vi "FFT Symbolic.vi"() -> ()   [LabVIEW 2020]
doc: "Calculates the Fourier transform for a symbolic equation that is entered on the front panel."
uses:
  <vilib>/Analysis/2dsp.llb/Real FFT.vi
  <vilib>/gmath/NI_Gmath.lvlib
  <vilib>/Analysis/NI_AALPro.lvlib
panel:
  in  "Tab Control":enum32{"Background", "Example"}(tab)
  out "OK":bool
  in  "Signal Type":u16(ring) items=["Square", "Sine", "Complex", "Arbitrary"]
  out "Response":cluster{"X Values":dbl[], "Y Values":dbl[]}[](graph)
  in  "function":string="square(x)-0.5"
  in  "order":i32(slide)=25 scale=0.0..100.0
  in  "Stop":bool
  # "Overview: Calculates the Fourier transform for a symbolic equation.\nRequirements: LabVIEW Full Development System\nInstructions:\n1. Run the VI and select the Example tab.\n2. Change the Signal Type and verify how this affects the response of the signal.\n3. Increase the order to see how the Gibbs Phenomena influences the signal.\n4. Click Stop to stop the VI."
  # "Gibbs Phenomenon"
  # "Fourier series 5th order"
  # "Fourier series 25th order"
  # "Fourier series can approximate any periodic function.\nThe more elements the better the approximation. The example depicts the approximation of a step function. Certain overshoot values are not avoidable in the case of discontinuous functions."
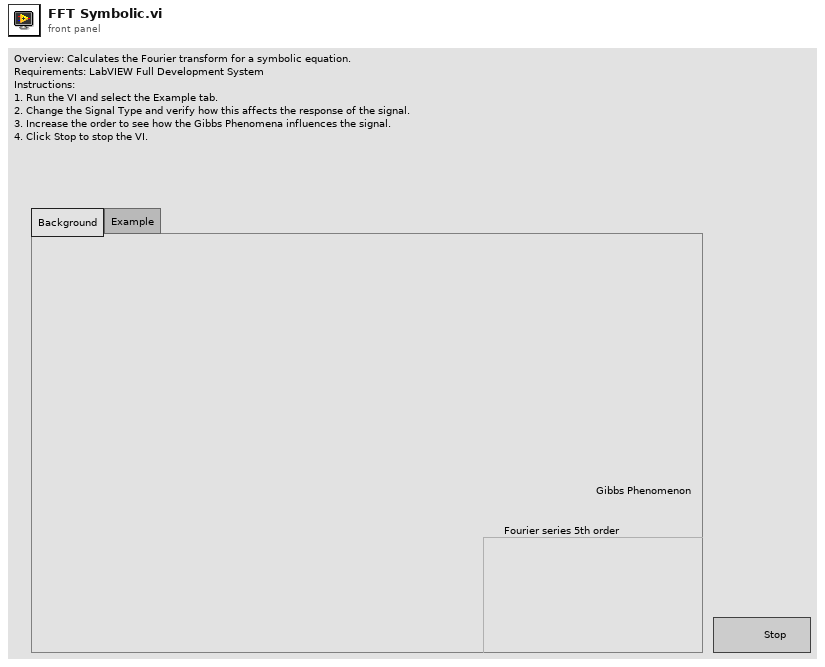
[diagram p1: front panel]
types:
  T1 = enum8{"Enabled", "Disabled", "Disabled and Grayed Out"}
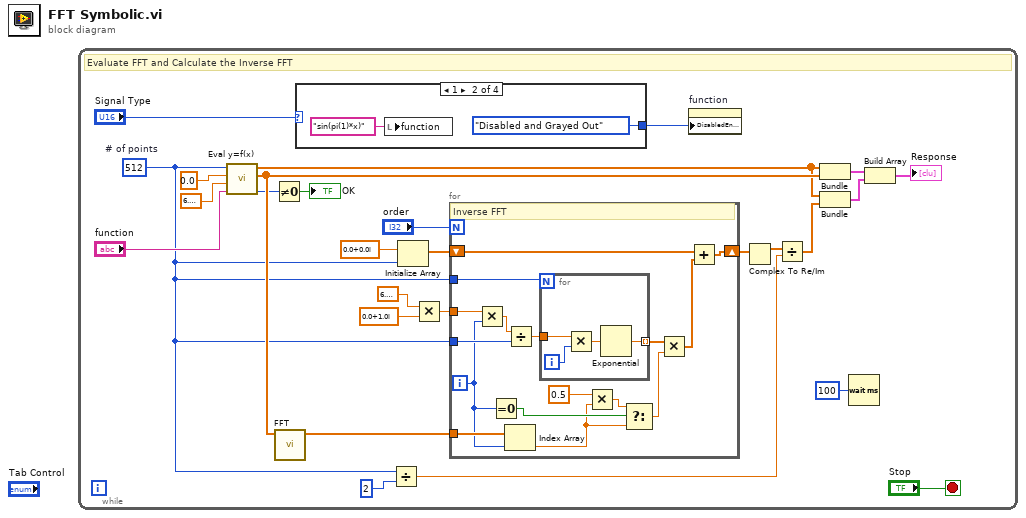
[diagram p0: block diagram]
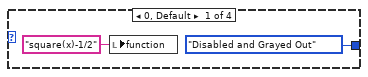
[diagram p2: hidden frame]
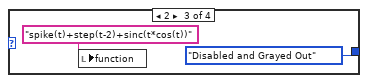
[diagram p3: hidden frame]
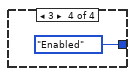
[diagram p4: hidden frame]
diagram:
  n1 = while {
    stop <- "Stop" stop-if-true
    w11 = 512  # # of points
    # "Evaluate FFT and Calculate the Inverse FFT"
    n2 = call <vilib>:"Eval y=f(x).vi"("formula"="function", "end"=6.283185307179586, "start"=0.0, "number of points"=w11) -> ("error"=w7:i32, "Y Values"=w26:dbl[], "X Values"=w19:dbl[])  [unwired: 1 out]
    n3 = Not Equal To 0?(x=w7) -> (x != 0?=→"OK":bool)
    n4 = call-poly <vilib>:"FFT.vi"("X"=w26) -> ("FFT {X}"=w20:cdb[])  [unwired: 2 in, 8 out]
    n5 = case shown="1" "Signal Type" {
      tunnel: [T1."Disabled and Grayed Out" ("Disabled") T1."Disabled and Grayed Out" ("Disabled") T1."Disabled and Grayed Out" ("Disabled") T1."Enabled" ("Disabled")] -> w5
      frame 0, Default {
        n6 = local write "function"("square(x)-1/2" ("function")) -> ()
      }
      frame 1 {
        n7 = local write "function"("sin(pi(1)*x)" ("function")) -> ()
      }
      frame 2 {
        n8 = local write "function"("spike(t)+step(t-2)+sinc(t*cos(t))" ("function")) -> ()
      }
      frame 3 {
      }
    }
    n9 = Divide(x=w11, y=2) -> (x/y=w15:dbl)
    n10 = Initialize Array(cdb 0.0+0.0i, w11) -> (w25:cdb[])
    n11 = Multiply(x=6.283185307179586, y=cdb 0.0+1.0i) -> (x*y=w17:cdb)
    n12 = for {
      N: "order" -> [_]
      shift-right: [w35] -> w21
      shift-left: w25 -> [w50]
      tunnel: w20 -> [w39]
      tunnel: w11 -> [w46]
      tunnel: w11 -> [w45]
      tunnel: w17 -> [w44]
      i -> [w38]
      # "Inverse FFT"
      n13 = Multiply(x=w44, y=w38) -> (x*y=w48:cdb)
      n14 = Equal To 0?(x=w38) -> (x = 0?=w42:bool)
      n15 = Index Array(array=w39, index=w38) -> (element=w37:cdb)
      n16 = Divide(x=w48, y=w46) -> (x/y=w47:cdb)
      n17 = for {
        N: w45 -> [_]
        tunnel: w47 -> [w53]
        tunnel: [w54] -> w40 mode=indexing
        i -> [w52]
        n18 = Multiply(x=w53, y=w52) -> (x*y=w51:cdb)
        n19 = Exponential(1:w51) -> (0:w54:cdb)
      }
      n20 = Multiply(x=0.5, y=w37) -> (x*y=w41:cdb)
      n21 = Select(t=w41, s=w42, f=w37) -> (s? t:f=w43:cdb)
      n22 = Multiply(x=w40, y=w43) -> (x*y=w49:cdb[])
      n23 = Add(x=w50, y=w49) -> (x+y=w35:cdb[])
    }
    n24 = property on="function" class="Str"("DisabledEnum"=w5) -> ()  [unwired: 2 in, 2 out]
    n25 = Complex To Re/Im(x + iy=w21) -> (x=w16:dbl[])  [unwired: 1 out]
    n26 = Divide(x=w16, y=w15) -> (x/y=w14:dbl[])
    n27 = Bundle("X Values"=w19, "Y Values"=w26) -> (w23:cluster{"X Values":dbl[], "Y Values":dbl[]})  [unwired: 1 out]
    n28 = Bundle("X Values"=w19, w14) -> (w22:cluster{"X Values":dbl[], dbl[]})  [unwired: 1 out]
    n29 = Wait (ms)(milliseconds to wait=u32 100) -> ()  [unwired: 1 out]
    n30 = Build Array(w23, w22) -> (→"Response":cluster{"X Values":dbl[], "Y Values":dbl[]}[])
  }
